vi "Calculate Port.vi"(8 "error in (no error)":errorcluster, 11 "TCP Listener in":refnum<class "TCP Listener.lvclass">) -> (0 "error out":errorcluster, 2 "Port":u16, 3 "TCP Listener out":refnum<class "TCP Listener.lvclass">)   [LabVIEW 2026, in "TALOS.lvlib" / "TCP Listener.lvlib" / "TCP Listener.lvclass"]
uses:
  TCP Listener.lvclass
  C:/LabVIEW Code/TALOS/talos/Ancestor/Ancestor/Ancestor.lvclass
  Ancestor/Ancestor/Ancestor.lvclass/Ancestor.ctl
  <vilib>/AdvancedString/Delimited String to 1D String Array (string).vi
  <vilib>/Utility/error.llb/Trim Whitespace (string).vi
  21389c36-1540-40d7-ab45-7d6bd8d23792.vi
  f84f0d72-010e-4fac-bce0-0d63b895174d.vi
  6e75f81f-6a96-418e-b5fe-5c4339ae1318.vi
  Ancestor/Ancestor/Read ID.vi
  Support VIs/Circus Config Param - Core.vi
  <vilib>/Utility/error.llb/Trim Whitespace One-Sided.vi
  f84f0d72-010e-4fac-bce0-0d63b895174d.vi/d4db2432-cc9c-482c-8957-dac855435ef6.vi
  f84f0d72-010e-4fac-bce0-0d63b895174d.vi/86fbf154-bd7b-49a2-8ab2-a837b2a95f24.vi
  f84f0d72-010e-4fac-bce0-0d63b895174d.vi/3b95b01e-1ec2-4565-bcd9-7606a5281010.vi
  f84f0d72-010e-4fac-bce0-0d63b895174d.vi/96a08935-737a-44b2-979c-a81d56408f7e.vi
  6e75f81f-6a96-418e-b5fe-5c4339ae1318.vi/d4db2432-cc9c-482c-8957-dac855435ef6.vi
  6e75f81f-6a96-418e-b5fe-5c4339ae1318.vi/86fbf154-bd7b-49a2-8ab2-a837b2a95f24.vi
  6e75f81f-6a96-418e-b5fe-5c4339ae1318.vi/3b95b01e-1ec2-4565-bcd9-7606a5281010.vi
  6e75f81f-6a96-418e-b5fe-5c4339ae1318.vi/96a08935-737a-44b2-979c-a81d56408f7e.vi
  Support VIs/Generate Error.vi
  Support VIs/Circus Root Path.vi
  Support VIs/TALOS Config Param.vi
  f84f0d72-010e-4fac-bce0-0d63b895174d.vi/d4db2432-cc9c-482c-8957-dac855435ef6.vi/6eaecd13-6e48-4772-a921-b51ebdf84d88.vi
  f84f0d72-010e-4fac-bce0-0d63b895174d.vi/d4db2432-cc9c-482c-8957-dac855435ef6.vi/d2d5f2b7-06f4-47f6-971c-049c3fdbb653.vi
  f84f0d72-010e-4fac-bce0-0d63b895174d.vi/3b95b01e-1ec2-4565-bcd9-7606a5281010.vi/6eaecd13-6e48-4772-a921-b51ebdf84d88.vi
  f84f0d72-010e-4fac-bce0-0d63b895174d.vi/3b95b01e-1ec2-4565-bcd9-7606a5281010.vi/d2d5f2b7-06f4-47f6-971c-049c3fdbb653.vi
  f84f0d72-010e-4fac-bce0-0d63b895174d.vi/96a08935-737a-44b2-979c-a81d56408f7e.vi/6eaecd13-6e48-4772-a921-b51ebdf84d88.vi
  f84f0d72-010e-4fac-bce0-0d63b895174d.vi/96a08935-737a-44b2-979c-a81d56408f7e.vi/d2d5f2b7-06f4-47f6-971c-049c3fdbb653.vi
  6e75f81f-6a96-418e-b5fe-5c4339ae1318.vi/d4db2432-cc9c-482c-8957-dac855435ef6.vi/6eaecd13-6e48-4772-a921-b51ebdf84d88.vi
  6e75f81f-6a96-418e-b5fe-5c4339ae1318.vi/d4db2432-cc9c-482c-8957-dac855435ef6.vi/d2d5f2b7-06f4-47f6-971c-049c3fdbb653.vi
  6e75f81f-6a96-418e-b5fe-5c4339ae1318.vi/3b95b01e-1ec2-4565-bcd9-7606a5281010.vi/6eaecd13-6e48-4772-a921-b51ebdf84d88.vi
  6e75f81f-6a96-418e-b5fe-5c4339ae1318.vi/3b95b01e-1ec2-4565-bcd9-7606a5281010.vi/d2d5f2b7-06f4-47f6-971c-049c3fdbb653.vi
  6e75f81f-6a96-418e-b5fe-5c4339ae1318.vi/96a08935-737a-44b2-979c-a81d56408f7e.vi/6eaecd13-6e48-4772-a921-b51ebdf84d88.vi
  6e75f81f-6a96-418e-b5fe-5c4339ae1318.vi/96a08935-737a-44b2-979c-a81d56408f7e.vi/d2d5f2b7-06f4-47f6-971c-049c3fdbb653.vi
  FGV/Error Memory/Get Error Description.vi
  Support VIs/Get PC name.vi
  Support VIs/Get Class Name.vi
  <vilib>/Utility/error.llb/Clear Errors.vi
  FGV/Error Memory/Error Memory Core.vi
  FGV/Error Memory/Error Crt Lvl checker.vi
  FGV/Error Memory/Error Memory Core.vi/40c8088d-b597-4017-91af-faa98e00292e.vi
  FGV/Error Memory/Error Memory Core.vi/d4a3ab98-063c-4e44-b43d-fbdcfe6c2be2.vi
  Support VIs/Global Constants.vi
  Support VIs/Global Memory.vi
  <vilib>/Utility/LVClass/Get LV Class Name.vi
  Support VIs/Is in Packed Library.vi
  Support VIs/TALOS Root path.vi
  Support VIs/Read CSV worksheet.vi
  <vilib>/Utility/error.llb/General Error Handler.vi
  <vilib>/Utility/config.llb/Open Config Data.vi
  <vilib>/Utility/config.llb/Get Section Names.vi
  <vilib>/Utility/config.llb/Get Key Names.vi
  <vilib>/Utility/config.llb/Read Key.vi
  <vilib>/Utility/config.llb/Read Key (String).vi
  <vilib>/Utility/config.llb/Close Config Data.vi
  Ancestor/Ancestor/Ancestor.lvclass
  <vilib>/Comparison/Equal/Equal Functor/Equal Functor.lvclass
  <vilib>/Comparison/Less/Less Functor/Less Functor.lvclass
  TALOS.lvlib
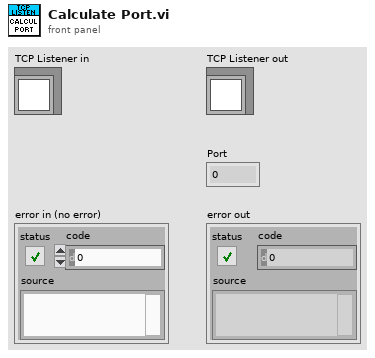
[diagram p1: front panel]
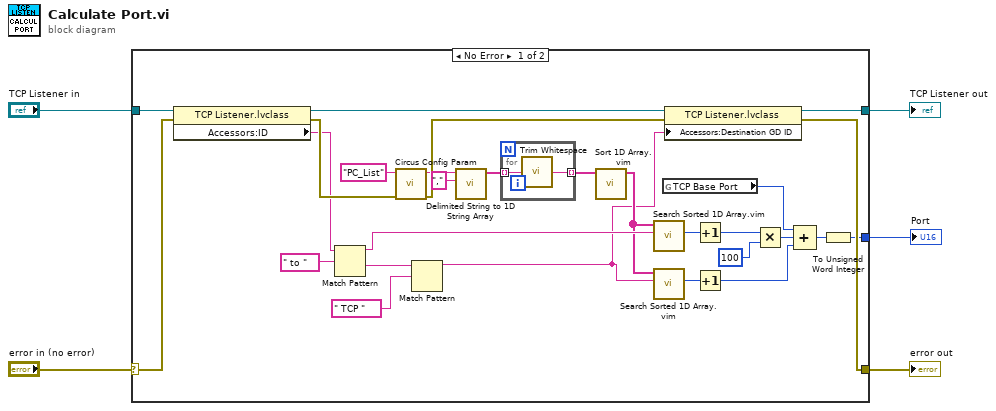
[diagram p0: block diagram]
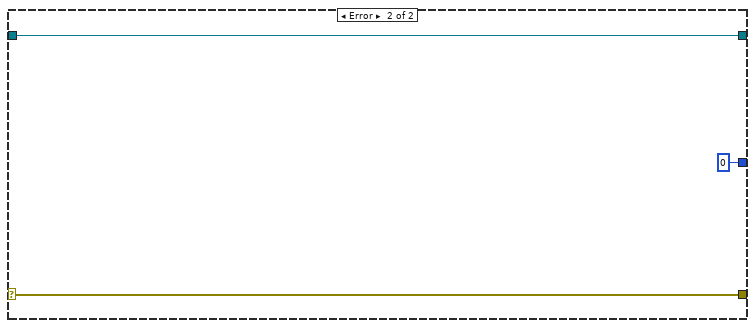
[diagram p2: hidden frame]
diagram:
  n1 = case shown="No Error" "error in (no error)" {
    selector: "error in (no error)" -> [w30 w36]
    tunnel: [w7 w38] -> w4
    tunnel: "TCP Listener in" -> [w28 w38]
    tunnel: [w8 u16 0] -> w2
    tunnel: [w33 w36] -> w1
    frame No Error {
      n2 = property class="TCP Listener.lvclass"(reference=w28, error in=w30) -> (reference out=w29:refnum<class "TCP Listener.lvclass">, error out=w31:errorcluster, "Accessors:ID"=w27:string)
      n3 = Match Pattern(string=w27, regular expression=" to " ("string")) -> (before substring=w18:string, after substring=w25:string)  [unwired: 1 in, 2 out]
      n4 = call "Circus Config Param.vi"("error in (no error)"=w31, "Parameter Name"="PC_List") -> ("error out"=w32:errorcluster, "Value"=w22:string)  [unwired: 8 in]
      n5 = Match Pattern(string=w25, regular expression=" TCP ") -> (before substring=w6:string)  [unwired: 1 in, 3 out]
      n6 = call-poly <vilib>:"Delimited String to 1D String Array.vi"("delimiter"=",", "delimited string"=w22) -> ("string array"=w20:string[])  [unwired: 9 in]
      n7 = for {
        tunnel: w20 -> [w35] mode=indexing
        tunnel: [w34] -> w19 mode=indexing
        n8 = call-poly <vilib>:"Trim Whitespace.vi"("string"=w35) -> ("trimmed string"=w34:string)  [unwired: 1 in]
      }
      n9 = call "Sort 1D Array.vim"("unsorted array"=w19) -> ("sorted array"=w17:string[])  [unwired: 10 in]
      n10 = call "Search Sorted 1D Array.vim"("element"=w18, "sorted 1D array"=w17) -> ("nearest index"=w16:i32)  [unwired: 8 in, 1 out]
      n11 = call "Search Sorted 1D Array.vim"("element"=w6, "sorted 1D array"=w17) -> ("nearest index"=w15:i32)  [unwired: 8 in, 1 out]
      n12 = global read "Global Constants.vi" "TCP Base Port"() -> (w12:u16)
      n13 = property class="TCP Listener.lvclass"(reference=w29, error in=w32, "Accessors:Destination GD ID"=w6) -> (reference out=w7:refnum<class "TCP Listener.lvclass">, error out=w33:errorcluster)
      n14 = Increment(x=w16) -> (x+1=w14:i32)
      n15 = Increment(x=w15) -> (x+1=w10:i32)
      n16 = Multiply(x=w14, y=u16 100) -> (x*y=w11:i32)
      n17 = Compound Arithmetic op=ADD(w12, w11, w10) -> (w9:i32)
      n18 = To Unsigned Word Integer(number=w9) -> (unsigned 16bit integer=w8:u16)
    }
    frame Error {
    }
  }
  "error out" <- w1
  "TCP Listener out" <- w4
  "Port" <- w2
